vi "FFOvl.vi"(0 "board_sel":u32=6) -> (1 "FFOvl 1":u8, 2 "FFOvl 2":u8)   [LabVIEW 2015]
uses:
  ESLSCDLL.dll
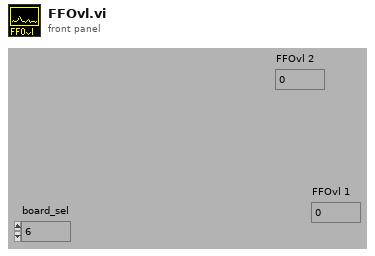
[diagram p1: front panel]
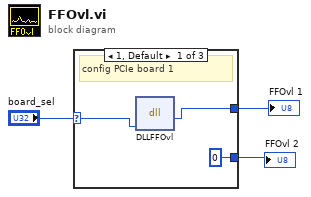
[diagram p0: block diagram]
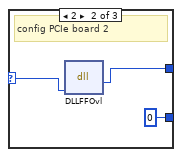
[diagram p2: hidden frame]
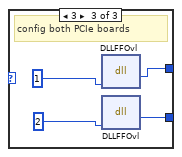
[diagram p3: hidden frame]
diagram:
  n1 = case shown="1, Default" "board_sel" {
    selector: "board_sel" -> [w6 w8 _]
    tunnel: [w5 w9 w11] -> w2
    tunnel: [u8 0 ("Rückgabetyp") u8 0 ("Rückgabetyp") w10] -> w1
    frame 1, Default {
      # "config PCIe board 1"
      n2 = dll-call lib="C:/Users/flori/Nextcloud/Dokumente/Stresing/Windows/lv64/board.vis/ESLSCDLL.dll" fn="DLLFFOvl"("drv"=w6) -> ("Rückgabetyp"=w5:u8)  [unwired: 4 in, 2 out]
    }
    frame 2 {
      # "config PCIe board 2"
      n3 = dll-call lib="C:/Users/flori/Nextcloud/Dokumente/Stresing/Windows/lv64/board.vis/ESLSCDLL.dll" fn="DLLFFOvl"("drv"=w8) -> ("Rückgabetyp"=w9:u8)  [unwired: 4 in, 2 out]
    }
    frame 3 {
      # "config both PCIe boards"
      n4 = dll-call lib="C:/Users/flori/Nextcloud/Dokumente/Stresing/Windows/lv64/board.vis/ESLSCDLL.dll" fn="DLLFFOvl"("drv"=u32 1) -> ("Rückgabetyp"=w11:u8)  [unwired: 4 in, 2 out]
      n5 = dll-call lib="C:/Users/flori/Nextcloud/Dokumente/Stresing/Windows/lv64/board.vis/ESLSCDLL.dll" fn="DLLFFOvl"("drv"=u32 2) -> ("Rückgabetyp"=w10:u8)  [unwired: 4 in, 2 out]
    }
  }
  "FFOvl 1" <- w2
  "FFOvl 2" <- w1
